vi "(SUBVI) - Read Light Sensor.vi"(8 "NXT/EV3":T2, 10 "Port (Port 1) 2":T1 items=["Port 1", "Port 2", "Port 3", "Port 4"], 11 "Port (Port 1)":T1 items=["Port 1", "Port 2", "Port 3", "Port 4"]) -> (0 "NXT/EV3 2":T2, 2 "Scaled Value 2":sgl, 3 "Scaled Value":sgl)   [LabVIEW 2016, in "testrobot.lvrbt"]
uses:
  testrobot.lvrbt
  <vilib>/NXT/Subs/LVHSConnector.ctl
  <vilib>/NXT/LegoClasses/BrickReference/BrickReference.lvclass
  <vilib>/NXT/Block Support/NXT_InputPort.ctl
  <vilib>/NXT/Dual Mode Library/Sensors/EV3_Color_Reflect.vi
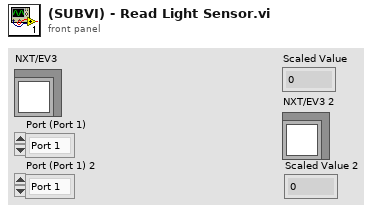
[diagram p1: front panel]
types:
  T1 = typedef "NXT_InputPort.ctl" = u32
  T2 = typedef "LVHSConnector.ctl" = refnum<class "BrickReference.lvclass">
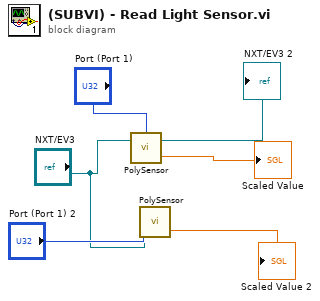
[diagram p0: block diagram]
diagram:
  n1 = call-poly <vilib>:"PolySensor.vi"("NXT/EV3"="NXT/EV3", "Port (Port 1)"="Port (Port 1)") -> ("Scaled Value"=→"Scaled Value":sgl, "NXT/EV3"=→"NXT/EV3 2":T2)  [unwired: 1 in]
  n2 = call-poly <vilib>:"PolySensor.vi"("NXT/EV3"="NXT/EV3", "Port (Port 1)"="Port (Port 1) 2") -> ("Scaled Value"=→"Scaled Value 2":sgl)  [unwired: 1 in, 1 out]
